vi "Get DataRow.vi"   [LabVIEW 2016, in "DataGrid.lvlib" / "DataGridView.lvclass"]
uses:
  <userlib>/LabVIEWdotNetDataGrid/source/DataGridView/DataGridView.lvclass
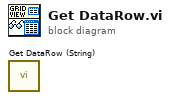
[diagram p0: block diagram]
diagram:
  n1 = call <userlib>:"Get DataRow (String).vi"() -> ()  [unwired: 9 in, 3 out]
